vi "Configure Thermistor.vi"(0 "VISA resource name":refnum<visa-resource-name>, 1 "Thermistor Type (ohms) (5000)":i32=5000, 5 "error in (no error)":errorcluster, 6 "Scan List (Empty)":string) -> (14 "VISA resource name out":refnum<visa-resource-name>, 19 "error out":errorcluster)   [LabVIEW 2020, in "Keithley 27XX.lvlib"]
doc: "This VI sets the transducer type to Thermistor. It also provided for configuration of a thermistor measurement.\n\nNote: \n(1) Configure Measurement.vi must be called <B>before</B> configuring the thermistor.\n\n(2) This VI will only work if the DMM is in Temperature Measurement mode.\n\n(3) The thermistor is a temperature sensitive resistor. Its resistance changes non-linearly with changes in temperature. Most thermistors have a negative temperature coefficient. As temperature increases, the resistance decreases. The DMM measures the resistance of the thermistor and calculates the temperature reading.\n\nOf all of the temperatrue transducers, the thermistor is the most sensitive. It can quickly detect minute changes in temperature. It is a good choice when measureing very small changes in temperature. The downside for the increased sensitivity is the loss of linearity. Since they are especially non-linear at high temperatures, it is best to use them for measurements below 100 deg C.\n\n(4) Temperature is calculated using the Steinhart-Hart equation."
uses:
  <instrlib>/Keithley 27XX/Keithley 27XX.lvlib
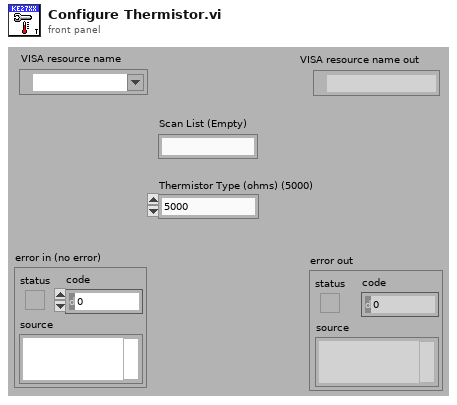
[diagram p1: front panel]
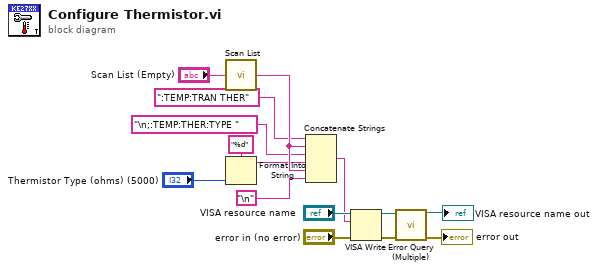
[diagram p0: block diagram]
diagram:
  n1 = call <instrlib>:"Scan List.vi"("Scan List (Empty)"="Scan List (Empty)") -> ("Scan List Out"=w15:string)  [unwired: 14 in]
  n2 = Format Into String(format string="%d", "Thermistor Type (ohms) (5000)") -> (resulting string=w7:string)  [unwired: 2 in, 1 out]
  n3 = Concatenate Strings(":TEMP:TRAN THER", w15, "\n;:TEMP:THER:TYPE ", w7, w15, "\n") -> (w12:string)
  n4 = VISA Write(VISA resource name="VISA resource name", write buffer=w12, error in (no error)="error in (no error)") -> (VISA resource name out=w5:refnum<visa-resource-name>, error out=w4:errorcluster)  [unwired: 1 out]
  n5 = call <instrlib>:"Error Query (Multiple).vi"("VISA resource name"=w5, "error in (no error)"=w4) -> ("VISA resource name out"=→"VISA resource name out":refnum<visa-resource-name>, "error out"=→"error out":errorcluster)  [unwired: 10 in, 2 out]
